vi "Initialise Multicol pair.vi"(10 "Calibration params listbox":refnum<vi>, 11 "Imaging params Listbox":refnum<vi>) -> ()   [LabVIEW 2020, in "MulColLBTable-pair.lvclass"]
uses:
  MulColLBTable-pair.lvclass
  MulColLBTable/MulColLBTable.lvclass
panel:
  out "Multicol-pair":refnum<class "MulColLBTable-pair.lvclass">
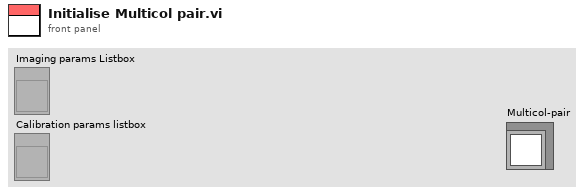
[diagram p1: front panel]
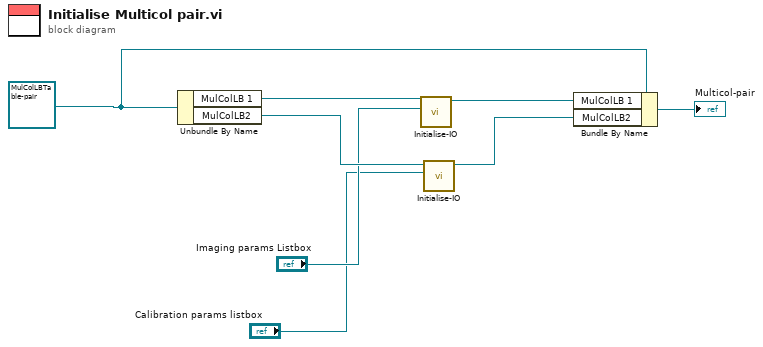
[diagram p0: block diagram]
diagram:
  w4 = refnum<class "MulColLBTable-pair.lvclass"> refnum ("MulColLBTable-pair.lvclass")
  n1 = Unbundle By Name(w4) -> ("MulColLB 1"=w8:refnum<class "MulColLBTable.lvclass">, "MulColLB2"=w7:refnum<class "MulColLBTable.lvclass">)
  n2 = call "Initialise-IO.vi"("Multicolumn Listbox"="Imaging params Listbox", "MulColLBTable.lvclass"=w8) -> ("MulColLBTable.lvclass out"=w3:refnum<class "MulColLBTable.lvclass">)  [unwired: 8 in, 1 out]
  n3 = call "Initialise-IO.vi"("Multicolumn Listbox"="Calibration params listbox", "MulColLBTable.lvclass"=w7) -> ("MulColLBTable.lvclass out"=w2:refnum<class "MulColLBTable.lvclass">)  [unwired: 8 in, 1 out]
  n4 = Bundle By Name(cluster=w4, "MulColLB 1"=w3, "MulColLB2"=w2) -> (→"Multicol-pair":refnum<class "MulColLBTable-pair.lvclass">)
